vi "Begin.vi"() -> (0 "error out":errorcluster)   [LabVIEW 2013, in "VirtualRobot.lvlib"]
uses:
  VirtualRobot.lvlib
  Systems/Driver/Driver.lvclass
  Systems/DriverTrain/DriveTrain.lvclass
  <vilib>/ActorFramework/Message Queue/Message Queue.lvclass/Message Queue.ctl
  Global Variables.vi
  <vilib>/ActorFramework/Actor/Actor.lvclass
  <vilib>/ActorFramework/Message Queue/Message Queue.lvclass
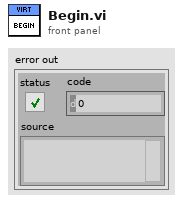
[diagram p1: front panel]
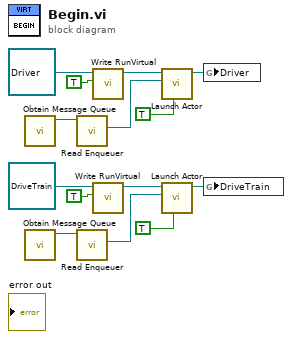
[diagram p0: block diagram]
diagram:
  n1 = call <vilib>:"Obtain Message Queue.vi"() -> ("Message Queue"=w14:refnum<class "Message Queue.lvclass">)  [unwired: 10 in, 1 out]
  n2 = call <vilib>:"Obtain Message Queue.vi"() -> ("Message Queue"=w5:refnum<class "Message Queue.lvclass">)  [unwired: 10 in, 1 out]
  n3 = call <vilib>:"Read Enqueuer.vi"("Message Queue"=w14) -> ("Message Enqueuer"=w13:refnum<class "Message Enqueuer.lvclass">)  [unwired: 10 in]
  n4 = call <vilib>:"Read Enqueuer.vi"("Message Queue"=w5) -> ("Message Enqueuer"=w4:refnum<class "Message Enqueuer.lvclass">)  [unwired: 10 in]
  n5 = call-dynamic "Write RunVirtual.vi"("RunVirtual?"=TRUE, "Driver in"=refnum<class "Driver.lvclass"> refnum ("Driver.lvlib:Driver.lvclass")) -> ("Driver out"=w9:refnum<class "Driver.lvclass">)  [unwired: 8 in, 1 out]
  n6 = call-dynamic "Write RunVirtual.vi"("RunVirtual"=TRUE, "DriveTrain in"=refnum<class "DriveTrain.lvclass"> refnum ("DriveTrain.lvlib:DriveTrain.lvclass")) -> ("DriveTrain out"=w3:refnum<class "DriveTrain.lvclass">)  [unwired: 8 in, 1 out]
  n7 = call <vilib>:"Launch Actor.vi"("Open Actor Core front panel? (F)"=TRUE, "Actor-to-Caller Enqueuer"=w13, "Actor"=w9) -> ("Caller-To-Actor Enqueuer"=w11:refnum<class "Message Enqueuer.lvclass">)  [unwired: 7 in, 1 out]
  n8 = call <vilib>:"Launch Actor.vi"("Open Actor Core front panel? (F)"=TRUE, "Actor-to-Caller Enqueuer"=w4, "Actor"=w3) -> ("Caller-To-Actor Enqueuer"=w1:refnum<class "Message Enqueuer.lvclass">)  [unwired: 7 in, 1 out]
  n9 = global write "Global Variables.vi" "Driver"(w11) -> ()
  n10 = global write "Global Variables.vi" "DriveTrain"(w1) -> ()
